vi "ComparePrefSets.vi"(1 "Prefs B":T1, 2 "Prefs A":T1) -> (0 "PrefDiffersArray":bool[](array[boolean]))   [LabVIEW 2013, in "SetListPrefs.lvclass"]
uses:
  SetListPrefs.lvclass
  PrefCluster.ctl
  <vilib>/Utility/miscctls.llb/LVRectTypeDef.ctl
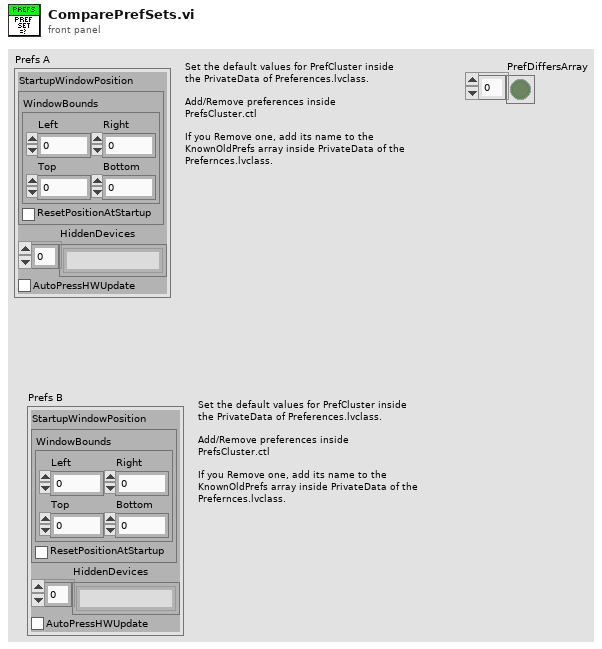
[diagram p1: front panel]
types:
  T1 = typedef "SetListPrefs.lvclass/PrefCluster.ctl" = cluster{"StartupWindowPosition":cluster{"WindowBounds":T2, "ResetPositionAtStartup":bool}, "HiddenDevices":string[], "AutoPressHWUpdate":bool}
  T2 = typedef "LVRectTypeDef.ctl" = cluster{"Left":i16, "Top":i16, "Right":i16, "Bottom":i16}
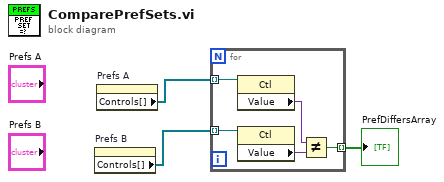
[diagram p0: block diagram]
diagram:
  n1 = property on="Prefs B" class="Clust (strict)"() -> ("Controls[]"=w1:refnum<vi>[])  [unwired: 2 in, 2 out]
  n2 = property on="Prefs A" class="Clust (strict)"() -> ("Controls[]"=w2:refnum<vi>[])  [unwired: 2 in, 2 out]
  n3 = for {
    tunnel: w2 -> [w8] mode=indexing
    tunnel: w1 -> [w7] mode=indexing
    tunnel: [w4] -> w3 mode=indexing
    n4 = property class="Ctl"(reference=w8) -> ("Value"=w5:variant)  [unwired: 1 in, 2 out]
    n5 = property class="Ctl"(reference=w7) -> ("Value"=w6:variant)  [unwired: 1 in, 2 out]
    n6 = Not Equal?(x=w5, y=w6) -> (x != y?=w4:bool)
  }
  "PrefDiffersArray" <- w3
